vi "Search Real Numbers without Approximation.vi"(11 "Complex Numbers In":cdb[](array[numeric])) -> (2 "Real Numbers":dbl[](array[numeric]), 3 "Complex Numbers Out":cdb[](array[numeric]))   [LabVIEW 2020, in "NI_AALPro.lvlib"]
uses:
  <vilib>/Analysis/NI_AALPro.lvlib
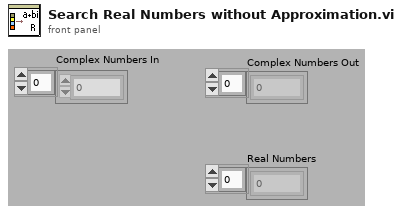
[diagram p1: front panel]
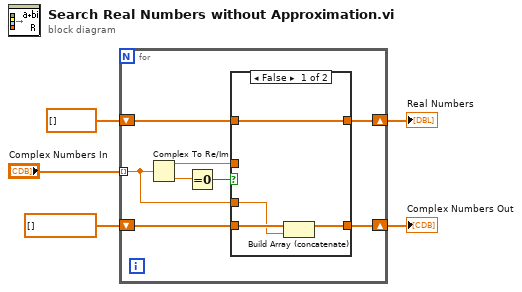
[diagram p0: block diagram]
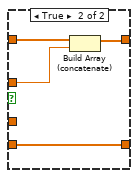
[diagram p2: hidden frame]
diagram:
  n1 = for {
    tunnel: "Complex Numbers In" -> [w9] mode=indexing
    shift-right: [w7] -> w2
    shift-left: dbl[] [] ("BDL") -> [w10]
    shift-right: [w6] -> w1
    shift-left: cdb[] [] ("CDB") -> [w11]
    n2 = Complex To Re/Im(x + iy=w9) -> (x=w8:dbl, y=w13:dbl)
    n3 = Equal To 0?(x=w13) -> (x = 0?=w12:bool)
    n4 = case shown="False" w12 {
      tunnel: w11 -> [w16 w18]
      tunnel: w10 -> [w17 w21]
      tunnel: w9 -> [w15 _]
      tunnel: w8 -> [_ w20]
      tunnel: [w17 w19] -> w7
      tunnel: [w14 w18] -> w6
      frame False {
        n5 = Build Array (concatenate)(w16, w15) -> (w14:cdb[])
      }
      frame True {
        n6 = Build Array (concatenate)(w21, w20) -> (w19:dbl[])
      }
    }
  }
  "Real Numbers" <- w2
  "Complex Numbers Out" <- w1
